vi "Practica 2 - Calculadora.vi"() -> ()   [LabVIEW 2023]
panel:
  out "DIVISION":dbl
  out "MULTIPLICACION":dbl
  out "RESTA":dbl
  out "SUMA":dbl
  in  "Y":dbl
  in  "X":dbl
  # "OPERACIONES BASICAS"
  # "Datos de entrada"
  # "Resultado"
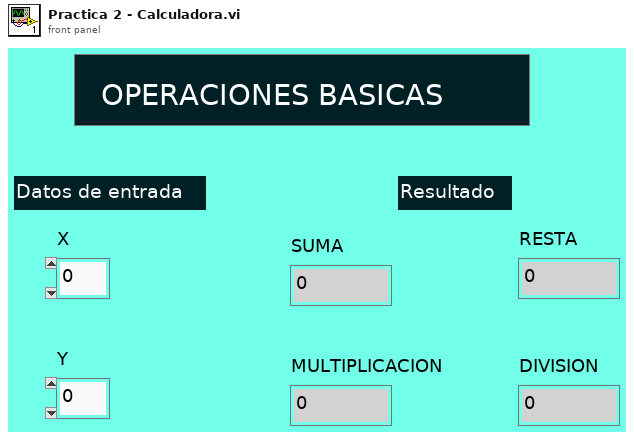
[diagram p1: front panel]
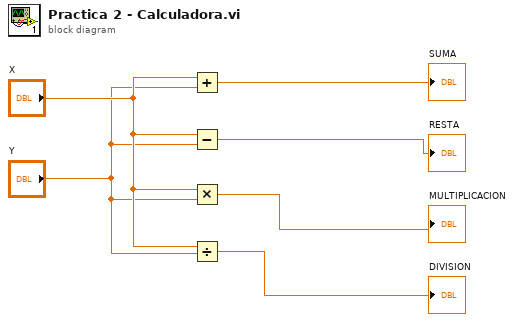
[diagram p0: block diagram]
diagram:
  n1 = Add(x="X", y="Y") -> (x+y=→"SUMA":dbl)
  n2 = Subtract(x="X", y="Y") -> (x-y=→"RESTA":dbl)
  n3 = Multiply(x="X", y="Y") -> (x*y=→"MULTIPLICACION":dbl)
  n4 = Divide(x="X", y="Y") -> (x/y=→"DIVISION":dbl)
